vi "Reach_Target.vi"(0 "Target_Position":dbl, 1 "Maintain_Samples":i32=10, 5 "Current_Position":dbl, 7 "Scale_Factor":dbl, 9 "Acceptable_Range":dbl, 11 "Timeout (ms)":i32=2000, 12 "Reset":bool) -> (4 "Motor_Value":dbl, 6 "Reached":bool)   [LabVIEW 2016]
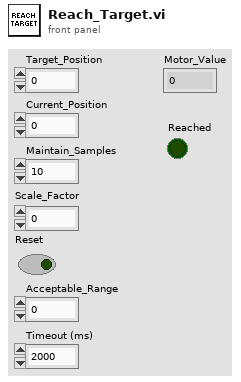
[diagram p1: front panel]
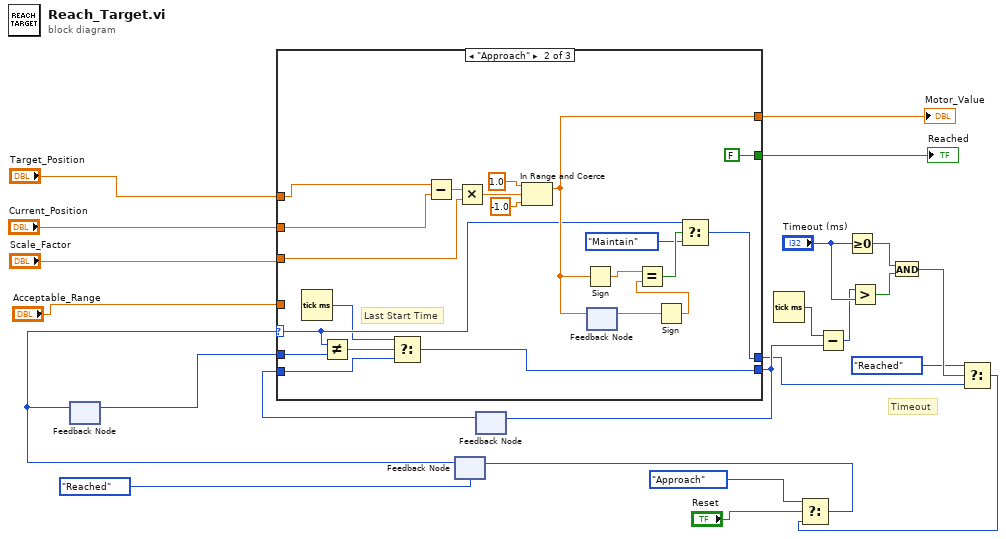
[diagram p0: block diagram]
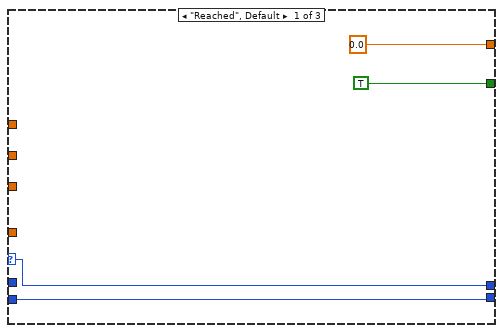
[diagram p2: hidden frame]
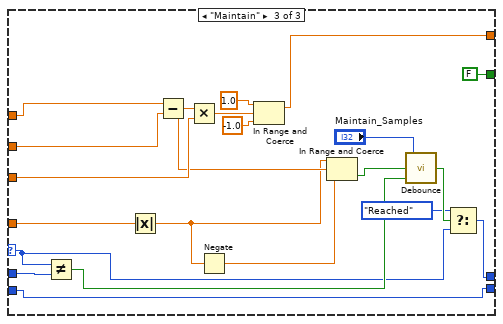
[diagram p3: hidden frame]
diagram:
  # "Timeout"
  n1 = feedback #1() -> (w12:enum16{"Reached", "Maintain", "Approach"})  [unwired: 1 in]
  n2 = feedback #2(enum16{"Reached", "Maintain", "Approach"}."Reached") -> (w13:enum16{"Reached", "Maintain", "Approach"})
  n3 = feedback-in #1(w13) -> ()
  n4 = feedback #3() -> (w11:u32)  [unwired: 1 in]
  n5 = case shown="\"Approach\"" w13 {
    selector: w13 -> [w25 w33 w52]
    tunnel: [w25 w34 w50] -> w3
    tunnel: [0.0 ("Motor_Value") w39 w62] -> w22
    tunnel: [TRUE ("Reached") FALSE ("Reached") FALSE ("Reached")] -> w21
    tunnel: "Current_Position" -> [_ w45 w67]
    tunnel: "Target_Position" -> [_ w46 w68]
    tunnel: "Scale_Factor" -> [_ w47 w69]
    tunnel: "Acceptable_Range" -> [_ _ w60]
    tunnel: w12 -> [_ w32 w55]
    tunnel: [w24 w30 w49] -> w8
    tunnel: w11 -> [w24 w29 w49]
    frame "Reached", Default {
    }
    frame "Approach" {
      # "Last Start Time"
      n6 = Tick Count (ms)() -> (millisecond timer value=w28:u32)
      n7 = Not Equal?(x=w33, y=w32) -> (x != y?=w31:bool)
      n8 = Select(t=w28, s=w31, f=w29) -> (s? t:f=w30:u32)
      n9 = Subtract(x=w46, y=w45) -> (x-y=w48:dbl)
      n10 = Multiply(x=w48, y=w47) -> (x*y=w44:dbl)
      n11 = In Range and Coerce(upper limit=1.0, x=w44, lower limit=-1.0) -> (coerced(x)=w39:dbl)  [unwired: 1 out]
      n12 = Sign(1:w39) -> (0:w38:dbl)
      n13 = feedback-in #4(w39) -> ()
      n14 = feedback #4() -> (w40:dbl)  [unwired: 1 in]
      n15 = Sign(1:w40) -> (0:w37:dbl)
      n16 = Equal?(x=w38, y=w37) -> (x = y?=w36:bool)
      n17 = Select(t=w33, s=w36, f=enum16{"Reached", "Maintain", "Approach"}."Maintain") -> (s? t:f=w34:enum16{"Reached", "Maintain", "Approach"})
    }
    frame "Maintain" {
      n18 = Not Equal?(x=w52, y=w55) -> (x != y?=w54:bool)
      n19 = Absolute Value(x=w60) -> (abs(x)=w59:dbl)
      n20 = Subtract(x=w68, y=w67) -> (x-y=w61:dbl)
      n21 = Multiply(x=w61, y=w69) -> (x*y=w66:dbl)
      n22 = Negate(x=w59) -> (-x=w58:dbl)
      n23 = In Range and Coerce(upper limit=1.0, x=w66, lower limit=-1.0) -> (coerced(x)=w62:dbl)  [unwired: 1 out]
      n24 = In Range and Coerce(upper limit=w59, x=w61, lower limit=w58) -> (In Range?=w57:bool)  [unwired: 1 out]
      n25 = call "Debounce.vi"("Reset"=w54, "Input"=w57, "Num samples"="Maintain_Samples") -> ("Output"=w53:bool)
      n26 = Select(t=enum16{"Reached", "Maintain", "Approach"}."Reached", s=w53, f=w52) -> (s? t:f=w50:enum16{"Reached", "Maintain", "Approach"})
    }
  }
  "Motor_Value" <- w22
  "Reached" <- w21
  n27 = feedback-in #3(w8) -> ()
  n28 = Tick Count (ms)() -> (millisecond timer value=w9:u32)
  n29 = Subtract(x=w9, y=w8) -> (x-y=w7:u32)
  n30 = Greater Or Equal To 0?(x="Timeout (ms)") -> (x >= 0?=w6:bool)
  n31 = Greater?(x=w7, y="Timeout (ms)") -> (0:w5:bool)
  n32 = And(x=w6, y=w5) -> (x .and. y?=w4:bool)
  n33 = Select(t=enum16{"Reached", "Maintain", "Approach"}."Reached", s=w4, f=w3) -> (s? t:f=w2:enum16{"Reached", "Maintain", "Approach"})
  n34 = Select(t=enum16{"Reached", "Maintain", "Approach"}."Approach", s="Reset", f=w2) -> (s? t:f=w19:enum16{"Reached", "Maintain", "Approach"})
  n35 = feedback-in #2(w19) -> ()
